vi "Build DashBoard Data.vi"(11 "Dashboard Enables":T3={"Analog Module 1"=[TRUE, TRUE, TRUE, TRUE, TRUE, TRUE, TRUE, TRUE], "Analog Module 2"=[FALSE, FALSE, FALSE, FALSE, FALSE, FALSE, FALSE, FALSE], "Digital Module 1"=TRUE, "Digital Module 2"=FALSE, "Solenoid Module"=TRUE}) -> ()   [LabVIEW 2011]
doc: "This VI builds data and sends it back to the dashboard PC program. By default it sends back the raw values for the first analog, digital, and solenoid module. Modify it to send back the data you want to view. Consider adding higher level data to the Dashboard Datatype.ctl and to this VI. Then update the Dashboard to display the data however you like.\n\nThis software is licensed. Open the labview\\readme\\WPI Robotics Library Open Source License.txt file for more information."
uses:
  DashboardEnable.ctl
  Dashboard Datatype.ctl
  <vilib>/Rock Robotics/WPI/DriverStation/WPI_DriverStationDigitalData.ctl
  Robot Global Data.vi
panel:
  out "Dashboard Data":T1 {"Left Drive" scale=0.0..10.0; "Right Drive" scale=0.0..10.0; "Shooter Speed" scale=0.0..10.0}
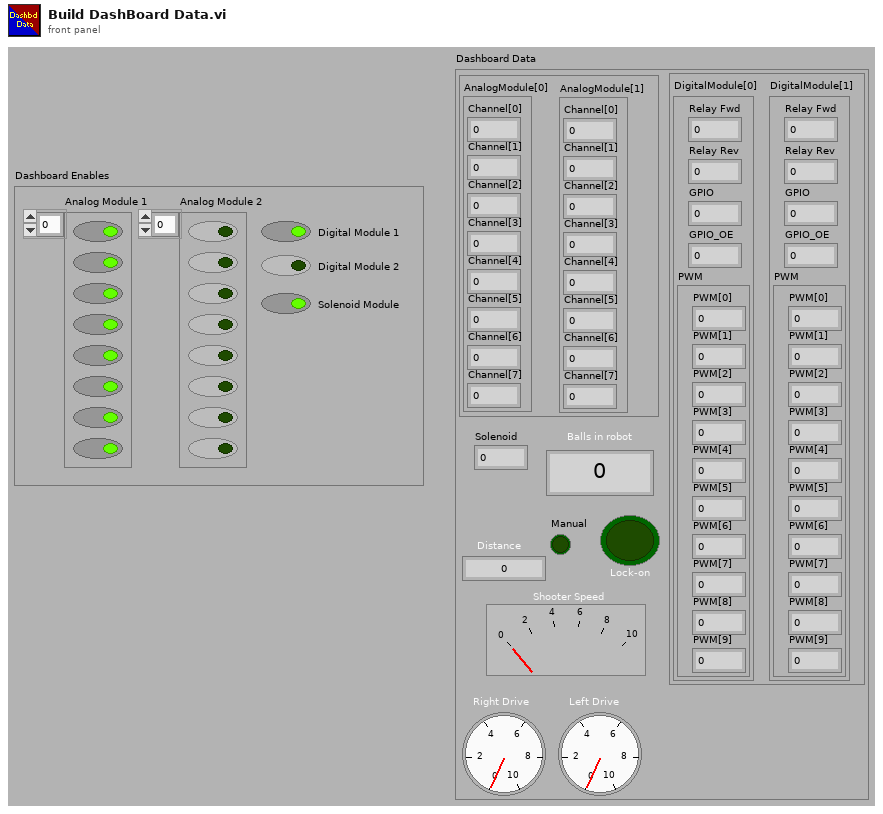
[diagram p1: front panel]
types:
  T1 = typedef "Dashboard Datatype.ctl" = cluster{cluster{"AnalogModule[0]":cluster{"Channel[0]":sgl, "Channel[1]":sgl, "Channel[2]":sgl, "Channel[3]":sgl, "Channel[4]":sgl, "Channel[5]":sgl, "Channel[6]":sgl, "Channel[7]":sgl}, "AnalogModule[1]":cluster{"Channel[0]":sgl, "Channel[1]":sgl, "Channel[2]":sgl, "Channel[3]":sgl, "Channel[4]":sgl, "Channel[5]":sgl, "Channel[6]":sgl, "Channel[7]":sgl}}, cluster{"DigitalModule[0]":T2, "DigitalModule[1]":T2}, "Solenoid":u8, "Balls in robot":dbl, "Lock-on":bool, "Shooter Speed":dbl, "Right Drive":dbl, "Left Drive":dbl, "Distance":dbl, "Manual":bool}
  T2 = typedef "WPI_DriverStationDigitalData.ctl" = cluster{"Relay Fwd":u8, "Relay Rev":u8, "GPIO":u16, "GPIO_OE":u16, "PWM":cluster{"PWM[0]":u8, "PWM[1]":u8, "PWM[2]":u8, "PWM[3]":u8, "PWM[4]":u8, "PWM[5]":u8, "PWM[6]":u8, "PWM[7]":u8, "PWM[8]":u8, "PWM[9]":u8}}
  T3 = typedef "DashboardEnable.ctl" = cluster{"Analog Module 1":bool[], "Analog Module 2":bool[], "Digital Module 1":bool, "Digital Module 2":bool, "Solenoid Module":bool}
  T4 = cluster{"AnalogModule[0]":cluster{"Channel[0]":sgl, "Channel[1]":sgl, "Channel[2]":sgl, "Channel[3]":sgl, "Channel[4]":sgl, "Channel[5]":sgl, "Channel[6]":sgl, "Channel[7]":sgl}, "AnalogModule[1]":cluster{"Channel[0]":sgl, "Channel[1]":sgl, "Channel[2]":sgl, "Channel[3]":sgl, "Channel[4]":sgl, "Channel[5]":sgl, "Channel[6]":sgl, "Channel[7]":sgl}}
  T5 = cluster{"Channel[0]":sgl, "Channel[1]":sgl, "Channel[2]":sgl, "Channel[3]":sgl, "Channel[4]":sgl, "Channel[5]":sgl, "Channel[6]":sgl, "Channel[7]":sgl}[]
  T6 = cluster{"Channel[0]":sgl, "Channel[1]":sgl, "Channel[2]":sgl, "Channel[3]":sgl, "Channel[4]":sgl, "Channel[5]":sgl, "Channel[6]":sgl, "Channel[7]":sgl}
  T7 = cluster{"AnalogModule[0][0]":sgl, "AnalogModule[0][1]":sgl, "AnalogModule[0][2]":sgl, "AnalogModule[0][3]":sgl, "AnalogModule[0][4]":sgl, "AnalogModule[0][5]":sgl, "AnalogModule[0][6]":sgl, "AnalogModule[0][7]":sgl}
  T8 = cluster{"[0]":cluster{"Channel[0]":sgl, "Channel[1]":sgl, "Channel[2]":sgl, "Channel[3]":sgl, "Channel[4]":sgl, "Channel[5]":sgl, "Channel[6]":sgl, "Channel[7]":sgl}, "[1]":cluster{"Channel[0]":sgl, "Channel[1]":sgl, "Channel[2]":sgl, "Channel[3]":sgl, "Channel[4]":sgl, "Channel[5]":sgl, "Channel[6]":sgl, "Channel[7]":sgl}}
  T9 = cluster{"DigitalModule[0]":T2, "DigitalModule[1]":T2}
  T10 = typedef "FPGA_DIODevRef.ctl" = cluster{"DevStatus":errorcluster, "Module":T11}
  T11 = typedef "FPGA_TypedefDigitalModule.ctl" = enum16{"Digital Module 1", "Digital Module 2"}
  T12 = cluster{"[0]":u8, "[1]":u8, "[2]":u8, "[3]":u8, "[4]":u8, "[5]":u8, "[6]":u8, "[7]":u8, "[8]":u8, "[9]":u8}
  T13 = typedef "FPGA_SolenoidDevRef.ctl" = cluster{"DevStatus":errorcluster, "Module":T14}
  T14 = typedef "FPGA_TypedefSolenoidModule.ctl" = enum16{"Solenoid Module 1", "Solenoid Module 2"}
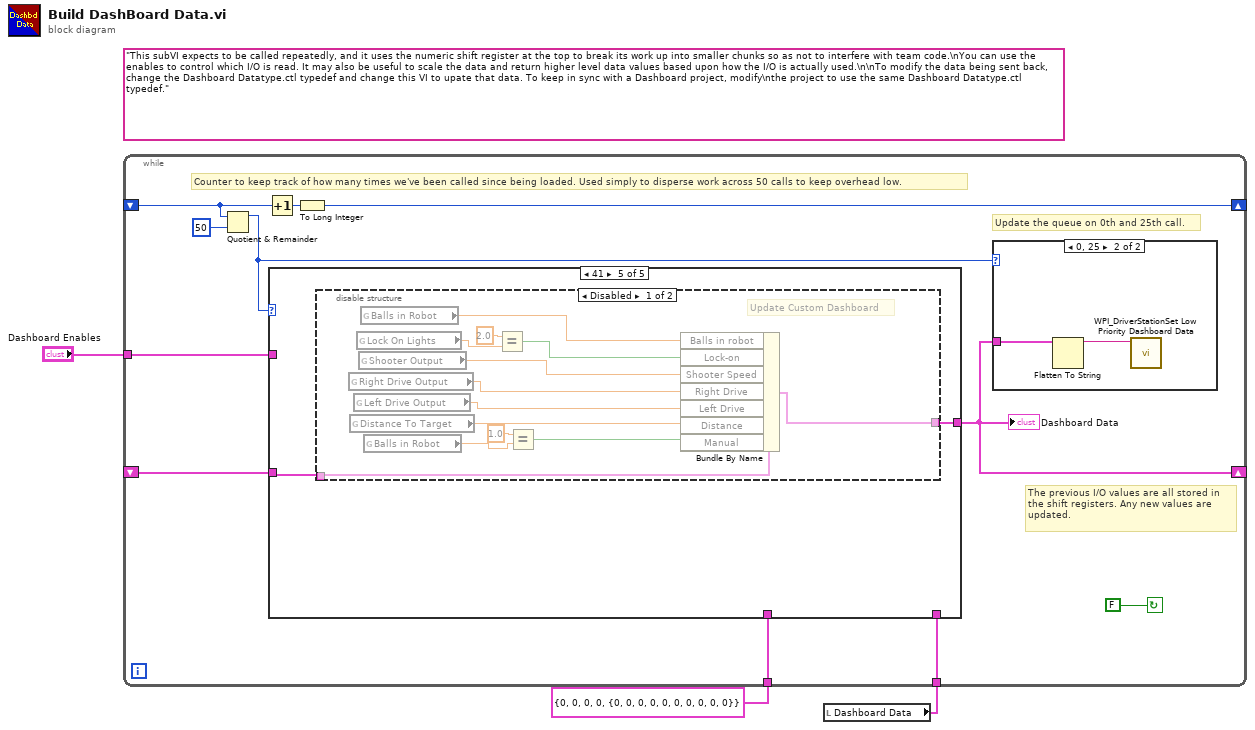
[diagram p0: block diagram]
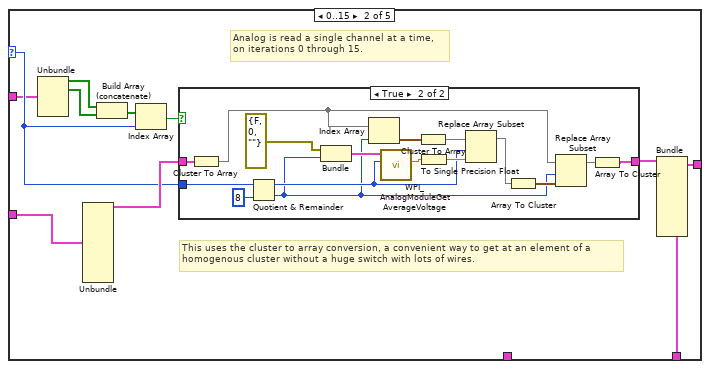
[diagram p4: hidden frame]
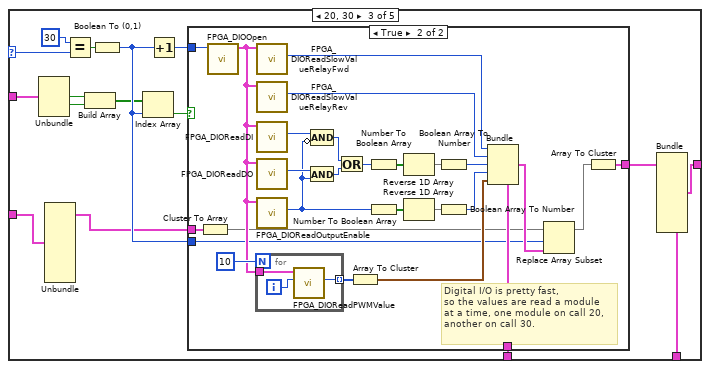
[diagram p6: hidden frame]
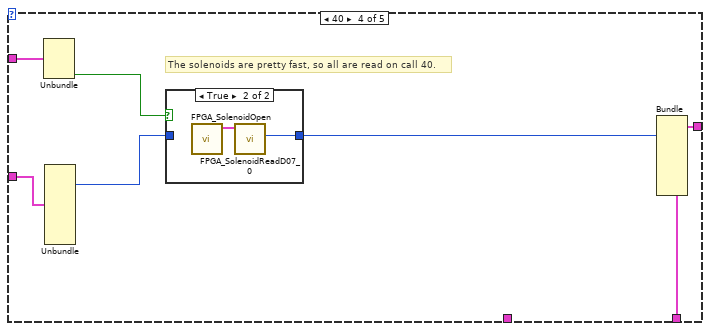
[diagram p8: hidden frame]
diagram:
  (unwired) "This subVI expects to be called repeatedly, and it uses the numeric shift register at the top to break its work up into smaller chunks so as not to interfere with team code.\nYou can use the enables to control which I/O is read. It may also be useful to scale the data and return higher level data values based upon how the I/O is actually used.\n\nTo modify the data being sent back, change the Dashboard Datatype.ctl typedef and change this VI to upate that data. To keep in sync with a Dashboard project, modify\nthe project to use the same Dashboard Datatype.ctl typedef."
  n1 = local read "Dashboard Data"() -> (w2:T1)
  n2 = while {
    shift-right: [w7] -> _
    shift-left: _ -> [w9]
    shift-right: [w4] -> _
    shift-left: _ -> [w12]
    tunnel: T2 {"Relay Fwd"=0, "Relay Rev"=0, "GPIO"=0, "GPIO_OE"=0, "PWM"={"PWM[0]"=0, "PWM[1]"=0, "PWM[2]"=0, "PWM[3]"=0, "PWM[4]"=0, "PWM[5]"=0, "PWM[6]"=0, "PWM[7]"=0, "PWM[8]"=0, "PWM[9]"=0}} ("DigitalModule[1]") -> [w11]
    tunnel: w2 -> [w6]
    tunnel: "Dashboard Enables" -> [w5]
    stop <- FALSE continue-if-true
    # "Counter to keep track of how many times we've been called since being loaded. Used simply to disperse work across 50 calls to keep overhead low."
    # "Update the queue on 0th and 25th call."
    # "The previous I/O values are all stored in\nthe shift registers. Any new values are\nupdated."
    n3 = Quotient & Remainder(x=w9, y=50) -> (x-y*floor(x/y)=w8:i32)  [unwired: 1 out]
    n4 = Increment(x=w9) -> (x+1=w14:i32)
    n5 = case shown="41" w8 {
      selector: w8 -> [_ w23 w55 _ _]
      tunnel: [w17 w19 w46 w95 w102] -> w4
      tunnel: w12 -> [w17 w18 w48 w97 w103]
      tunnel: w11 -> [_ _ w61 _ _]
      tunnel: w6 -> [_ w25 w47 w94 _]
      tunnel: w5 -> [_ w22 w53 w98 _]
      frame Default {
        # "Don't update any I/O"
      }
      frame 0..15 {
        # "This uses the cluster to array conversion, a convenient way to get at an element of a\nhomogenous cluster without a huge switch with lots of wires."
        # "Analog is read a single channel at a time,\non iterations 0 through 15."
        n6 = Unbundle(w22) -> ("Analog Module 1"=w21:bool[], "Analog Module 2"=w20:bool[])  [unwired: 3 out]
        n7 = Unbundle(w18) -> (w24:T4)  [unwired: 9 out]
        n8 = Build Array (concatenate)(w21, w20) -> (w27:bool[])
        n9 = Index Array(array=w27, index=w23) -> (element=w28:bool)
        n10 = case shown="True" w28 {
          tunnel: w23 -> [_ w36]
          tunnel: [w29 w33] -> w26
          tunnel: w24 -> [w29 w32]
          frame False {
          }
          frame True {
            n11 = Cluster To Array(cluster=w32) -> (array=w31:T5)
            n12 = Quotient & Remainder(x=w36, y=8) -> (x-y*floor(x/y)=w35:i32, floor(x/y)=w30:i32)
            n13 = Bundle("DevStatus"=errorcluster {"status"=FALSE, "code"=0, "source"=""}, w30) -> (w44:cluster{"DevStatus":errorcluster, i32})  [unwired: 1 out]
            n14 = Index Array(array=w31, index=w30) -> (element=w38:T6)
            n15 = call <vilib>:"WPI_AnalogModuleGetAverageVoltage.vi"("Channel"=w35, "AnalogModuleDevStatus"=w44) -> ("Average Voltage"=w41:dbl)  [unwired: 1 in, 8 out]
            n16 = Cluster To Array(cluster=w38) -> (array=w37:sgl[])
            n17 = To Single Precision Float(number=w41) -> (single precision float=w40:sgl)
            n18 = Replace Array Subset(array=w37, new element=w40, index=w35) -> (w39:sgl[])
            n19 = Array To Cluster(array=w39) -> (cluster=w43:T7)
            n20 = Replace Array Subset(array=w31, new element=w43, index=w30) -> (w34:T5)
            n21 = Array To Cluster(array=w34) -> (cluster=w33:T8)
          }
        }
        n22 = Bundle(cluster=w25, w26) -> (w19:T1)  [unwired: 9 out]
      }
      frame 20, 30 {
        n23 = Unbundle(w53) -> ("Digital Module 1"=w52:bool, "Digital Module 2"=w51:bool)  [unwired: 3 out]
        n24 = Unbundle(w48) -> (w50:T9)  [unwired: 9 out]
        n25 = Equal?(x=30, y=w55) -> (x = y?=w59:bool)
        n26 = Build Array(w52, w51) -> (w54:bool[])
        n27 = Boolean To (0,1)(Boolean=w59) -> (0, 1=w57:i16)
        n28 = Index Array(array=w54, index=w57) -> (element=w56:bool)
        n29 = Increment(x=w57) -> (x+1=w58:i16)
        n30 = case shown="True" w56 {
          tunnel: w61 -> [_ w70]
          tunnel: [w62 w63] -> w49
          tunnel: w58 -> [_ w68]
          tunnel: w57 -> [_ w67]
          tunnel: w50 -> [w62 w66]
          frame False {
          }
          frame True {
            # "Digital I/O is pretty fast,\nso the values are read a module\nat a time, one module on call 20,\nanother on call 30."
            n31 = Cluster To Array(cluster=w66) -> (array=w65:T2[])
            n32 = call <vilib>:"FPGA_DIOOpen.vi"("Module (Module 1)"=w68) -> ("DIODeviceRef"=w86:T10)  [unwired: 1 in, 9 out]
            n33 = for {
              N: 10 -> [_]
              tunnel: w86 -> [w91]
              tunnel: [w89] -> w87 mode=indexing
              i -> [w90]
              n34 = call <vilib>:"FPGA_DIOReadPWMValue.vi"("PWMChannel"=w90, "DIODeviceRef In"=w91) -> ("PWMValue"=w89:u8)  [unwired: 1 in, 8 out]
            }
            n35 = call <vilib>:"FPGA_DIOReadSlowValueRelayFwd.vi"("DIODeviceRef In"=w86) -> ("Relay Forward"=w79:u8)  [unwired: 1 in, 9 out]
            n36 = call <vilib>:"FPGA_DIOReadSlowValueRelayRev.vi"("DIODeviceRef In"=w86) -> ("Relay Reverse"=w80:u8)  [unwired: 1 in, 9 out]
            n37 = call <vilib>:"FPGA_DIOReadDI.vi"("DIODeviceRef In"=w86) -> ("DI"=w84:u16)  [unwired: 1 in, 9 out]
            n38 = call <vilib>:"FPGA_DIOReadDO.vi"("DIODeviceRef In"=w86) -> ("DO"=w83:u16)  [unwired: 1 in, 9 out]
            n39 = call <vilib>:"FPGA_DIOReadOutputEnable.vi"("DIODeviceRef In"=w86) -> ("OutputEnable"=w74:u16)  [unwired: 1 in, 9 out]
            n40 = And(x=w83, y=w74) -> (x .and. y?=w82:u16)
            n41 = Compound Arithmetic op=AND(w84, invert w74) -> (w81:u16)
            n42 = Or(x=w81, y=w82) -> (x .or. y?=w72:u16)
            n43 = Array To Cluster(array=w87) -> (cluster=w85:T12)
            n44 = Number To Boolean Array(number=w72) -> (Boolean array=w77:bool[])
            n45 = Number To Boolean Array(number=w74) -> (Boolean array=w76:bool[])
            n46 = Reverse 1D Array(array=w77) -> (reversed array=w78:bool[])
            n47 = Reverse 1D Array(array=w76) -> (reversed array=w75:bool[])
            n48 = Boolean Array To Number(Boolean array=w78) -> (number=w71:u32)
            n49 = Boolean Array To Number(Boolean array=w75) -> (number=w73:u32)
            n50 = Bundle(cluster=w70, "Relay Fwd"=w79, "Relay Rev"=w80, "GPIO"=w71, "GPIO_OE"=w73, "PWM"=w85) -> (w69:T2)
            n51 = Replace Array Subset(array=w65, new element=w69, index=w67) -> (w64:T2[])
            n52 = Array To Cluster(array=w64) -> (cluster=w63:cluster{"[0]":T2, "[1]":T2})
          }
        }
        n53 = Bundle(cluster=w47, w49) -> (w46:T1)  [unwired: 9 out]
      }
      frame 40 {
        # "The solenoids are pretty fast, so all are read on call 40."
        n54 = Unbundle(w98) -> ("Solenoid Module"=w92:bool)  [unwired: 4 out]
        n55 = Unbundle(w97) -> ("Solenoid"=w96:u8)  [unwired: 9 out]
        n56 = case shown="True" w92 {
          tunnel: [w99 w100] -> w93
          tunnel: w96 -> [w99 _]
          frame False {
          }
          frame True {
            n57 = call <vilib>:"FPGA_SolenoidOpen.vi"() -> ("SolenoidDevRef"=w101:T13)  [unwired: 2 in, 9 out]
            n58 = call <vilib>:"FPGA_SolenoidReadD07_0.vi"("SolenoidDevRef"=w101) -> ("DO7:0"=w100:u8)  [unwired: 1 in, 9 out]
          }
        }
        n59 = Bundle(cluster=w94, "Solenoid"=w93) -> (w95:T1)  [unwired: 9 out]
      }
      frame 41 {
        n60 = disable-structure shown="Disabled" {
          disable-tunnel: w103 -> [w116 w117]
          disable-tunnel: [w115 w117] -> w102
          frame Disabled {
            # "Update Custom Dashboard"
            n61 = global read "Robot Global Data.vi" "Right Drive Output"() -> (w112:dbl)
            n62 = global read "Robot Global Data.vi" "Distance To Target"() -> (w113:dbl)
            n63 = global read "Robot Global Data.vi" "Left Drive Output"() -> (w111:dbl)
            n64 = global read "Robot Global Data.vi" "Lock On Lights"() -> (w110:dbl)
            n65 = global read "Robot Global Data.vi" "Shooter Output"() -> (w107:dbl)
            n66 = global read "Robot Global Data.vi" "Balls in Robot"() -> (w114:dbl)
            n67 = global read "Robot Global Data.vi" "Balls in Robot"() -> (w105:dbl)
            n68 = Equal?(x=2.0, y=w110) -> (x = y?=w108:bool)
            n69 = Equal?(x=1.0, y=w105) -> (x = y?=w104:bool)
            n70 = Bundle By Name(cluster=w116, "Balls in robot"=w114, "Lock-on"=w108, "Shooter Speed"=w107, "Right Drive"=w112, "Left Drive"=w111, "Distance"=w113, "Manual"=w104) -> (w115:T1)
          }
          frame Enabled {
          }
        }
      }
    }
    "Dashboard Data" <- w4
    n71 = To Long Integer(number=w14) -> (32bit integer=w7:i32)
    n72 = case shown="0, 25" w8 {
      tunnel: w4 -> [_ w16]
      frame Default {
      }
      frame 0, 25 {
        n73 = Flatten To String(anything=w16) -> (data string=w15:string)  [unwired: 1 in, 4 out]
        n74 = call <vilib>:"WPI_DriverStationSet Low Priority Dashboard Data.vi"("User Data"=w15) -> ()  [unwired: 1 in, 10 out]
      }
    }
  }
